vi "Update Last Time.vi"(8 "error in (no error)":errorcluster, 11 "[MV] Key Certify in":refnum<class "[MV] Key Certify.lvclass">) -> (0 "error out":errorcluster, 3 "[MV] Key Certify out":refnum<class "[MV] Key Certify.lvclass">)   [LabVIEW 2020, in "[MV] Key Certify.lvlib" / "[MV] Key Certify.lvclass"]
uses:
  [MV] Key Certify.lvclass
  <vilib>/registry/registry.llb/Registry RtKey.ctl
  <vilib>/registry/registry.llb/Write Registry Value Simple STR.vi
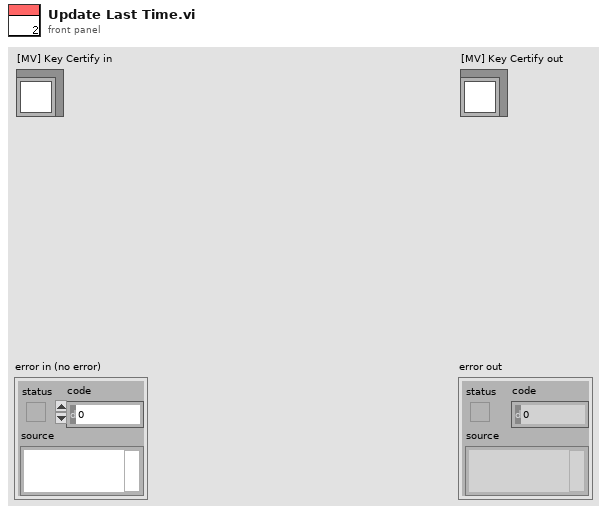
[diagram p1: front panel]
types:
  T1 = typedef "Registry RtKey.ctl" = enum32{"HKEY_CLASSES_ROOT", "HKEY_CURRENT_USER", "HKEY_LOCAL_MACHINE", "HKEY_USERS", "HKEY_PERFORMANCE_DATA", "HKEY_CURRENT_CONFIG", "HKEY_DYN_DATA"}
  T2 = typedef "Registry refnum.ctl" = refnum<k1>
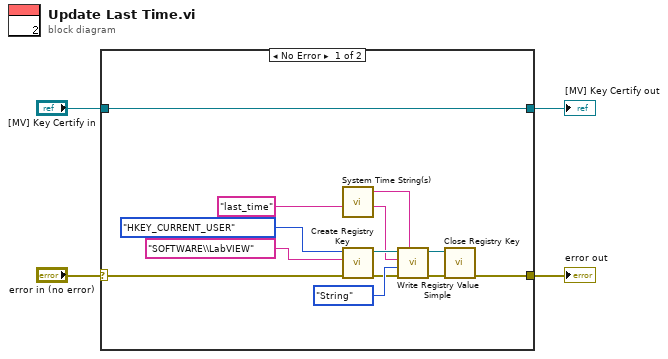
[diagram p0: block diagram]
diagram:
  n1 = case shown="No Error" "error in (no error)" {
    selector: "error in (no error)" -> [w6 w18]
    tunnel: [w5 w18] -> w3
    tunnel: [w16 w17] -> w1
    tunnel: "[MV] Key Certify in" -> [w16 w17]
    frame No Error {
      n2 = call <vilib>:"System Time String(s).vi"() -> ("system time string(s)"=w7:string)  [unwired: 5 in]
      n3 = call <vilib>:"Create Registry Key.vi"("error in (no error)"=w6, "subkey"="SOFTWARE\\LabVIEW", "root key (HKEY_LOCAL_MACHINE)"=Registry_RtKey."HKEY_CURRENT_USER") -> ("error out"=w11:errorcluster, "refnum out"=w12:T2)  [unwired: 6 in, 1 out]
      n4 = call-poly <vilib>:"Write Registry Value Simple.vi"("String/Binary data"=w7, "error in (no error)"=w11, "simple data type"=enum16{"String", "Binary", "DWORD"}."String", "value"="last_time" ("String/Binary data"), "refnum"=w12) -> ("error out"=w13:errorcluster, "refnum out"=w14:T2)  [unwired: 3 in]
      n5 = call <vilib>:"Close Registry Key.vi"("error in (no error)"=w13, "refnum"=w14) -> ("error out"=w5:errorcluster)  [unwired: 5 in]
    }
    frame Error {
    }
  }
  "error out" <- w3
  "[MV] Key Certify out" <- w1
